vi "WriterCore.vi"(0 "File Size":u32=2048 caption="File Size (internal)", 1 "Initiational":bool caption="Initiational (internal)", 2 "Close":bool caption="Close (internal)", 3 "Filename":string="hurricane.4pf" caption="Filename (internal)", 8 "NXT":T1={"Hardware"="NXT", "Flattened String"=""}) -> (11 "NXT":T1)   [LabVIEW 2010, in "Packet Recorder.lvlib"]
uses:
  Packet Recorder.lvlib
  <vilib>/NXT/Subs/LVHSConnector.ctl
  Remote Interface/Remote Interface.lvlib
panel:
  out "Stored Filename":string="hurricane.4pf"
  in  "stored loop index":u32
  out "stored timer value":u32
  out "Stored Joystick Data":string
  out "Stored Button Data":string
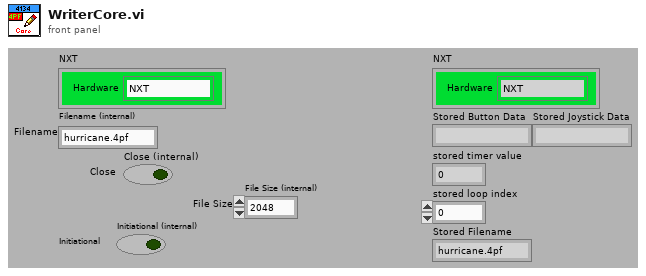
[diagram p1: front panel]
types:
  T1 = typedef "LVHSConnector.ctl" = cluster{"Hardware":string, "Flattened String":string}
  T2 = typedef "FTC ControllerState.ctl" = cluster{"Left X":i8, "Left Y":i8, "Right X":i8, "Right Y":i8, "Button Encoding 9-12":u8, "Button Encoding 1-8":u8, "POV":T3}
  T3 = typedef "FTC POVState.ctl" = i8
  T4 = cluster{"1B1-12:2B1-12:1POV:2POV":bool[], "1LXY:RXY:2LXY:RXY":bool[]}
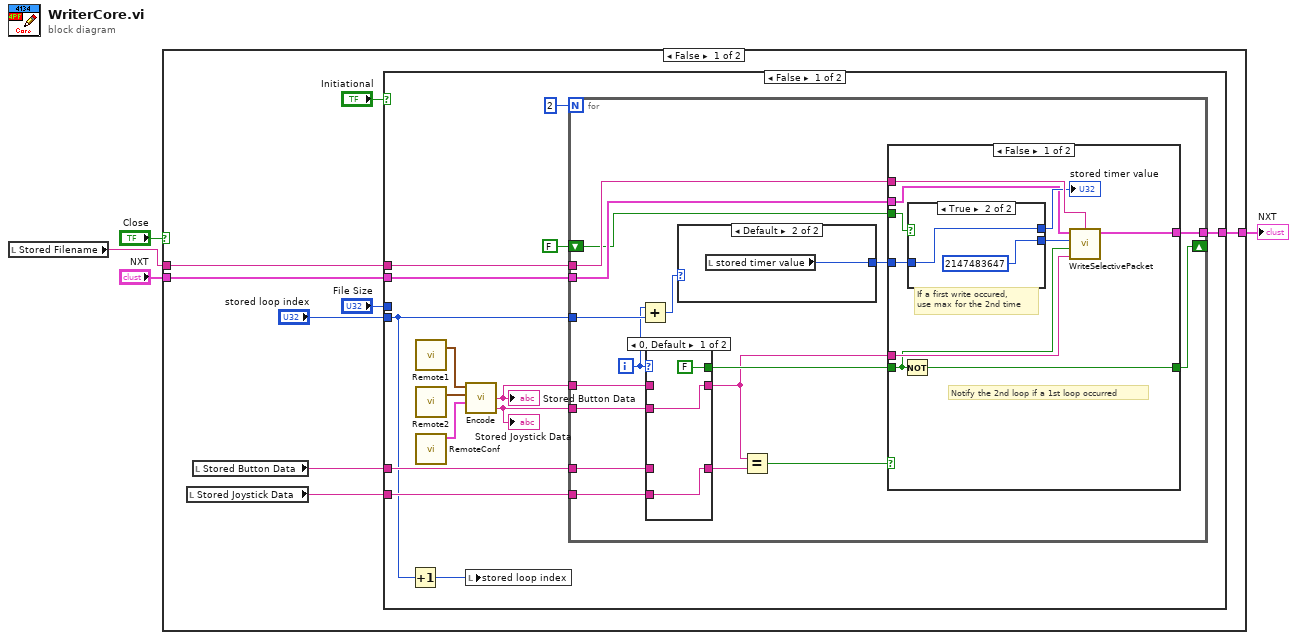
[diagram p0: block diagram]
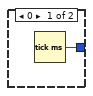
[diagram p2: hidden frame]
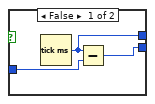
[diagram p3: hidden frame]
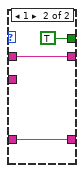
[diagram p5: hidden frame]
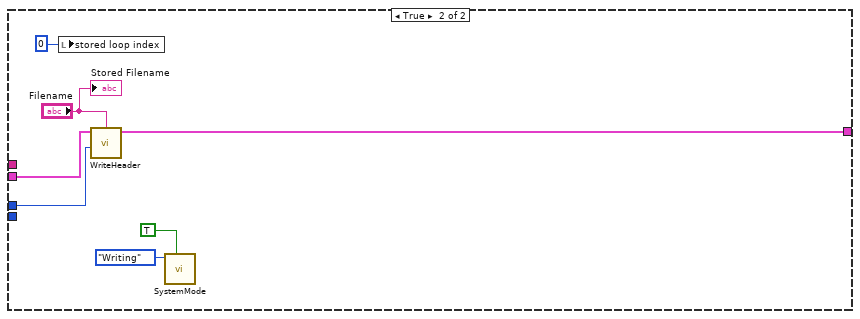
[diagram p6: hidden frame]
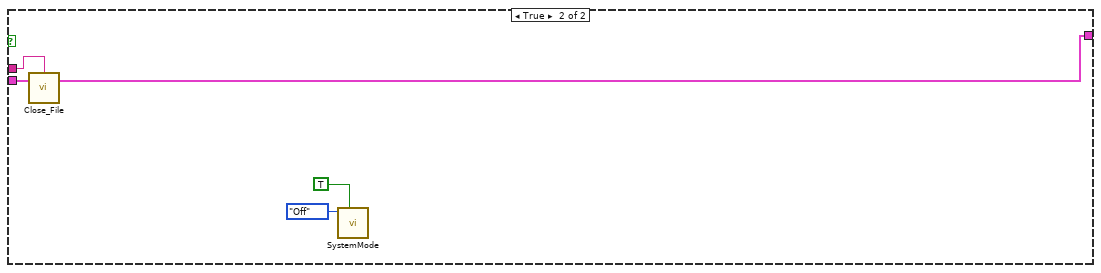
[diagram p7: hidden frame]
diagram:
  n1 = local read "Stored Filename"() -> (w3:string)
  n2 = case shown="False" "Close" {
    tunnel: "NXT" -> [w10 w78]
    tunnel: w3 -> [w7 w79]
    tunnel: [w5 w77] -> w2
    frame False {
      n3 = local read "Stored Joystick Data"() -> (w8:string)
      n4 = local read "Stored Button Data"() -> (w9:string)
      n5 = case shown="False" "Initiational" {
        tunnel: w7 -> [w17 _]
        tunnel: "File Size" -> [_ w73]
        tunnel: w10 -> [w15 w74]
        tunnel: w9 -> [w20 _]
        tunnel: w8 -> [w19 _]
        tunnel: "stored loop index" -> [w14 _]
        tunnel: [w16 w70] -> w5
        frame False {
          n6 = Increment(x=w14) -> (x+1=w18:u32)
          n7 = call "Remote1.vi"() -> ("Controller State"=w25:T2)  [unwired: 4 in]
          n8 = call "Remote2.vi"() -> ("Controller State"=w24:T2)  [unwired: 4 in]
          n9 = call "RemoteConf.vi"() -> ("Conf"=w26:T4)  [unwired: 11 in]
          n10 = call "Encode.vi"("Conf"=w26, "Controller 2 State"=w24, "Controller 1 State"=w25) -> ("Joystick Data"=w21:string, "Button Data"=w22:string)  [unwired: 2 in]
          "Stored Button Data" <- w22
          "Stored Joystick Data" <- w21
          n11 = local write "stored loop index"(w18) -> ()
          n12 = for {
            N: 2 -> [_]
            tunnel: w22 -> [w43]
            tunnel: w21 -> [w42]
            tunnel: w20 -> [w41]
            tunnel: w19 -> [w40]
            tunnel: w17 -> [w36]
            tunnel: [w34] -> w16
            tunnel: w15 -> [w33]
            tunnel: w14 -> [w32]
            shift-right: [w29] -> _
            shift-left: FALSE -> [w28]
            i -> [w30]
            n13 = Add(x=w30, y=w32) -> (x+y=w31:u32)
            n14 = case shown="0, Default" w30 {
              tunnel: w43 -> [_ w67]
              tunnel: w42 -> [w64 _]
              tunnel: w41 -> [_ w66]
              tunnel: w40 -> [w63 _]
              tunnel: [w64 w67] -> w35
              tunnel: [w63 w66] -> w39
              tunnel: [FALSE TRUE] -> w38
              frame 0, Default {
              }
              frame 1 {
              }
            }
            n15 = case shown="Default" w31 {
              tunnel: [w44 w45] -> w27
              frame 0 {
                n16 = Tick Count (ms)() -> (millisecond timer value=w44:u32)
              }
              frame Default {
                n17 = local read "stored timer value"() -> (w45:u32)
              }
            }
            n18 = Equal?(x=w35, y=w39) -> (x = y?=w37:bool)
            n19 = case shown="False" w37 {
              tunnel: w38 -> [w47 _]
              tunnel: w36 -> [w55 _]
              tunnel: w35 -> [w54 _]
              tunnel: w27 -> [w53 _]
              tunnel: [w51 w61] -> w34
              tunnel: w33 -> [w50 w61]
              tunnel: [w48 _] -> w29
              tunnel: w28 -> [w49 _]
              frame False {
                # "If a first write occured,\nuse max for the 2nd time"
                # "Notify the 2nd loop if a 1st loop occurred"
                n20 = Not(x=w47) -> (.not. x?=w48:bool)
                n21 = case shown="True" w49 {
                  tunnel: w53 -> [w58 w60]
                  tunnel: [w57 w60] -> w52
                  tunnel: [w56 2147483647 ("y")] -> w46
                  frame False {
                    n22 = Tick Count (ms)() -> (millisecond timer value=w57:u32)
                    n23 = Subtract(x=w57, y=w58) -> (x-y=w56:u32)
                  }
                  frame True {
                  }
                }
                "stored timer value" <- w52
                n24 = call "WriteSelectivePacket.vi"("Filename"=w55, "NXT"=w50, "Time (MS)"=w46, "F:Joysticks T:Buttons"=w47, "Encoded Data"=w54) -> ("NXT"=w51:T1)  [unwired: 4 in]
              }
              frame True {
              }
            }
          }
        }
        frame True {
          n25 = local write "stored loop index"(u32 0 ("stored loop index")) -> ()
          n26 = call "WriteHeader.vi"("Filename"="Filename", "NXT"=w74, "File Size (2048)"=w73) -> ("NXT"=w70:T1)  [unwired: 6 in]
          n27 = call "SystemMode.vi"("Write?"=TRUE, "ModeInput"=enum16{"Off", "Reading", "Writing"}."Writing") -> ()  [unwired: 9 in, 1 out]
          "Stored Filename" <- "Filename"
        }
      }
    }
    frame True {
      n28 = call <vilib>:"Close_File.vi"("NXT"=w78, "Filename"=w79) -> ("NXT"=w77:T1)  [unwired: 2 in]
      n29 = call "SystemMode.vi"("Write?"=TRUE, "ModeInput"=enum16{"Off", "Reading", "Writing"}."Off") -> ()  [unwired: 9 in, 1 out]
    }
  }
  "NXT" <- w2
